vi "create.vi"(7 "librarian_sm in":refnum<class "librarian.lvclass">, 8 "error in (no error)":errorcluster) -> (0 "error out":errorcluster, 3 "librarian_sm out":refnum<class "librarian.lvclass">)   [LabVIEW 2020, in "librarian.lvclass"]
uses:
  librarian.lvclass
  librarian.lvclass/librarian.ctl
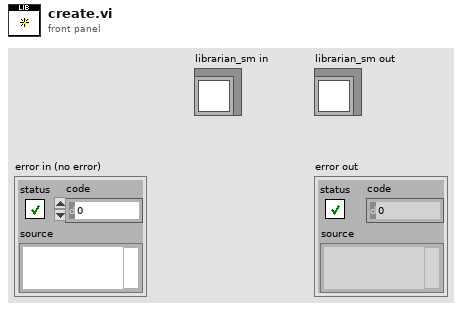
[diagram p1: front panel]
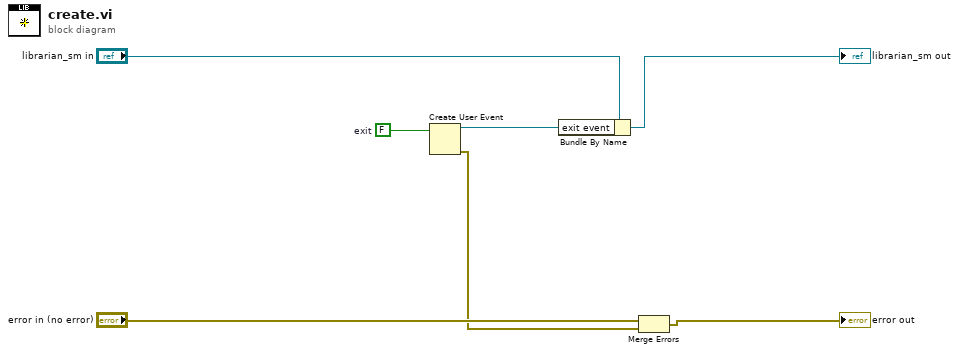
[diagram p0: block diagram]
diagram:
  w1 = FALSE  # exit
  n1 = Create User Event(user event datatype=w1) -> (user event=w5:refnum<user-event>, error out=w3:errorcluster)  [unwired: 1 in]
  n2 = Bundle By Name(cluster="librarian_sm in", "exit event"=w5) -> (→"librarian_sm out":refnum<class "librarian.lvclass">)
  n3 = Merge Errors("error in (no error)", w3) -> (→"error out":errorcluster)
